vi "Function_Generator.vi"() -> ()   [LabVIEW 2015]
panel:
  in  "Wave Type":enum16{"Triangle", "Sine", "Sawtooth", "Square"}(ring)
  out "Waveform Graph":dynamicdata(graph)
  in  "Frequency":i32
  in  "Amplitude":i32
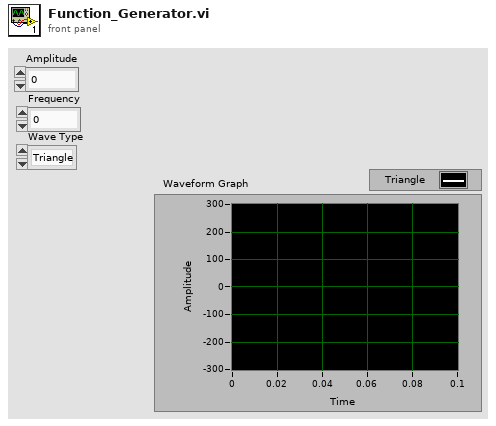
[diagram p1: front panel]
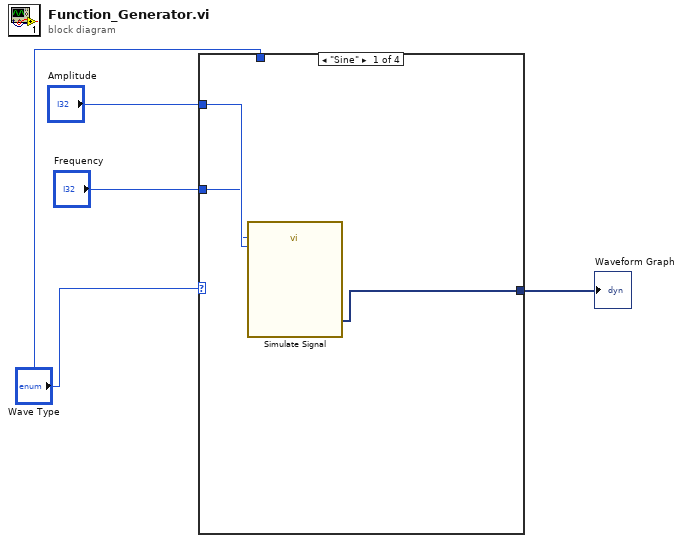
[diagram p0: block diagram]
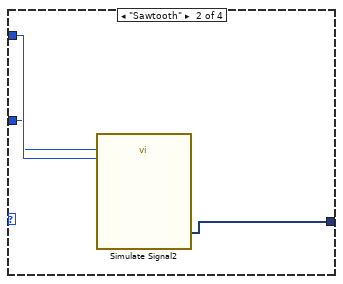
[diagram p2: hidden frame]
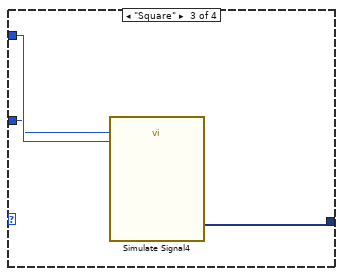
[diagram p3: hidden frame]
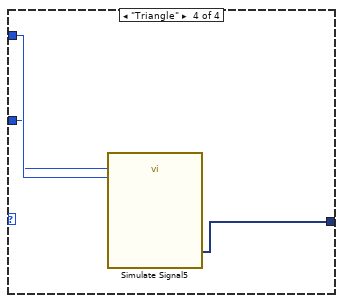
[diagram p4: hidden frame]
diagram:
  n1 = case shown="\"Sine\"" "Wave Type" {
    tunnel: "Amplitude" -> [w7 w10 w13 w16]
    tunnel: "Frequency" -> [w6 w9 w12 w15]
    tunnel: [w5 w8 w11 w14] -> w2
    tunnel: "Wave Type" -> [_ _ _ _]
    frame "Sine" {
      n2 = call "Simulate Signal"("Frequency"=w6, "Amplitude"=w7) -> ("Sine"=w5:dynamicdata)  [unwired: 12 in, 1 out]
    }
    frame "Sawtooth" {
      n3 = call "Simulate Signal2"("Frequency"=w9, "Amplitude"=w10) -> ("Sawtooth"=w8:dynamicdata)  [unwired: 12 in, 1 out]
    }
    frame "Square" {
      n4 = call "Simulate Signal4"("Frequency"=w12, "Amplitude"=w13) -> ("Square"=w11:dynamicdata)  [unwired: 12 in, 1 out]
    }
    frame "Triangle" {
      n5 = call "Simulate Signal5"("Frequency"=w15, "Amplitude"=w16) -> ("Triangle"=w14:dynamicdata)  [unwired: 12 in, 1 out]
    }
  }
  "Waveform Graph" <- w2
